vi "题目2.vi"() -> ()   [LabVIEW 2017]
panel:
  out "数值2":dbl
  out "数值":dbl
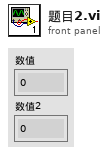
[diagram p1: front panel]
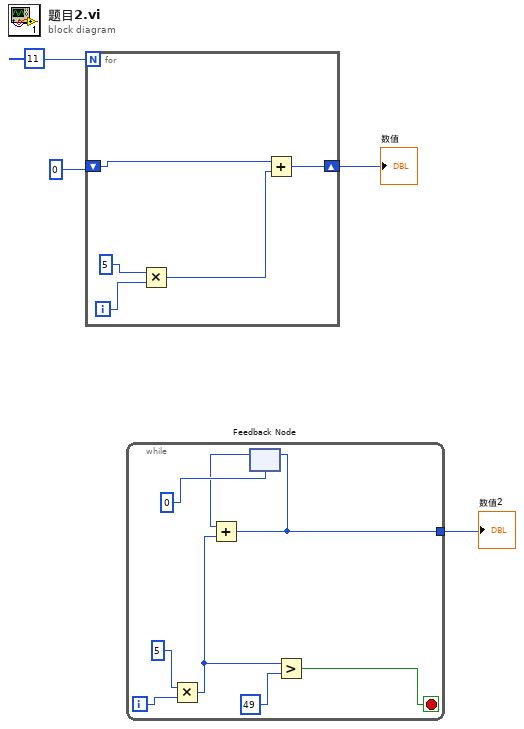
[diagram p0: block diagram]
diagram:
  n1 = for {
    N: 11 -> [_]
    shift-right: [w5] -> w3
    shift-left: 0 -> [w7]
    i -> [w8]
    n2 = Multiply(x=5, y=w8) -> (x*y=w6:i32)
    n3 = Add(x=w7, y=w6) -> (x+y=w5:i32)
  }
  "数值" <- w3
  n4 = while {
    tunnel: [w10] -> w1
    i -> [w14]
    stop <- w11 stop-if-true
    n5 = Multiply(x=5, y=w14) -> (x*y=w12:i32)
    n6 = feedback #1(0) -> (w16:i32)
    n7 = Add(x=w16, y=w12) -> (x+y=w10:i32)
    n8 = feedback-in #1(w10) -> ()
    n9 = Greater?(x=w12, y=49) -> (0:w11:bool)
  }
  "数值2" <- w1
